vi "Pre Launch Init.vi"(11 "Ancestor in":refnum<class "Ancestor.lvclass">) -> (0 "error out":errorcluster, 3 "Ancestor out":refnum<class "Ancestor.lvclass">)   [LabVIEW 2026, in "TALOS.lvlib" / "Ancestor.lvlib" / "Ancestor.lvclass"]
doc: "(<B>Filename</B>: Actor Framework.lvlib:Actor.lvclass:Pre Launch Init.vi)\n\nDefines behavior that occurs after the Launch Nested Actor method is invoked but before the actor's Actor Core method begins running.\n\nBy default, this method does nothing. A descendant class may override it to define behavior."
uses:
  Ancestor.lvclass
  Infinite Message Selector.ctl
  builds/Actor Framework PPL/Actor Framework.lvlibp/1abvi3w/vi.lib/ActorFramework/Actor/Actor.lvclass
  TALOS.lvlib
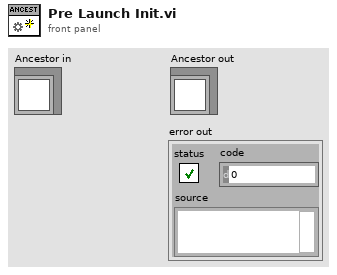
[diagram p1: front panel]
types:
  T1 = typedef "TALOS.lvlib/Ancestor.lvlib/Ancestor.lvclass/Infinite Message Selector.ctl" = enum16{"Start", "Stop", "Check", "Flush (Stop all)", "Init"}
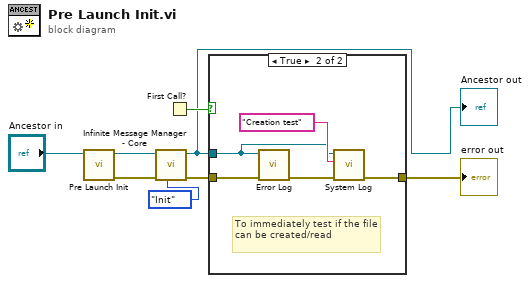
[diagram p0: block diagram]
diagram:
  n1 = call-parent "Pre Launch Init.vi"("Actor in"="Ancestor in") -> ("error out"=w5:errorcluster, "Actor out"=w6:refnum<class "Ancestor.lvclass">)  [unwired: 9 in]
  n2 = call-dynamic "Infinite Message Manager - Core.vi"("Infinite Message Selector"=Infinite_Message_Selector."Init", "error in (no error)"=w5, "Ancestor in"=w6) -> ("error out"=w2:errorcluster, "Ancestor out"=w1:refnum<class "Ancestor.lvclass">)  [unwired: 6 in, 1 out]
  "Ancestor out" <- w1
  n3 = First Call?() -> (First Call?: T/F=w4:bool)
  n4 = case shown="True" w4 {
    tunnel: [w9 w14] -> w7
    tunnel: w2 -> [w9 w12]
    tunnel: w1 -> [_ w10]
    frame False {
    }
    frame True {
      # "To immediately test if the file can be created/read"
      n5 = call "Error Log.vi"("error in (no error)"=w12, "Object in"=w10) -> ("error out"=w11:errorcluster)  [unwired: 9 in]
      n6 = call "System Log.vi"("error in (no error)"=w11, "Text to log"="Creation test", "Object in"=w10) -> ("error out"=w14:errorcluster)  [unwired: 8 in]
    }
  }
  "error out" <- w7
